vi "lvlib_copy.vi"(7 "configuration":T1={"project_file"="", "lvlibp_directory"="", "zip_directory"="", "lvlib_directory"="", "update_version_vi"="", "installer_post_file"="", "distribution_folder"="", "dependencies_folder"="", "version"="", "bin_folder"="", "lvlib_post_action"=0, "installer_post_action"=0, "application_post_action"=0, "zip_post_action"=1}, 8 "error in (no error)":errorcluster, 11 "library_path":path) -> (0 "error out":errorcluster, 3 "copied_library_path":path)   [LabVIEW 2015, in "lv-builder-default.lvlib"]
uses:
  lv-builder-default.lvlib
  public/_controls/configuration.ctl
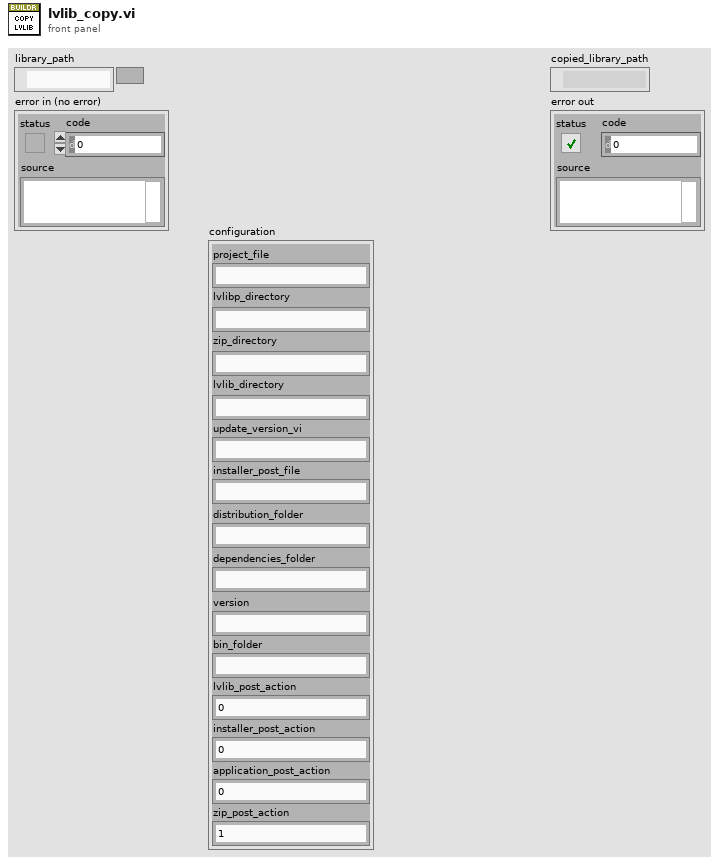
[diagram p1: front panel]
types:
  T1 = typedef "lv-builder-default.lvlib/configuration.ctl" = cluster{"project_file":string, "lvlibp_directory":string, "zip_directory":string, "lvlib_directory":string, "update_version_vi":string, "installer_post_file":string, "distribution_folder":string, "dependencies_folder":string, "version":string, "bin_folder":string, "lvlib_post_action":u16, "installer_post_action":u16, "application_post_action":u16, "zip_post_action":u16}
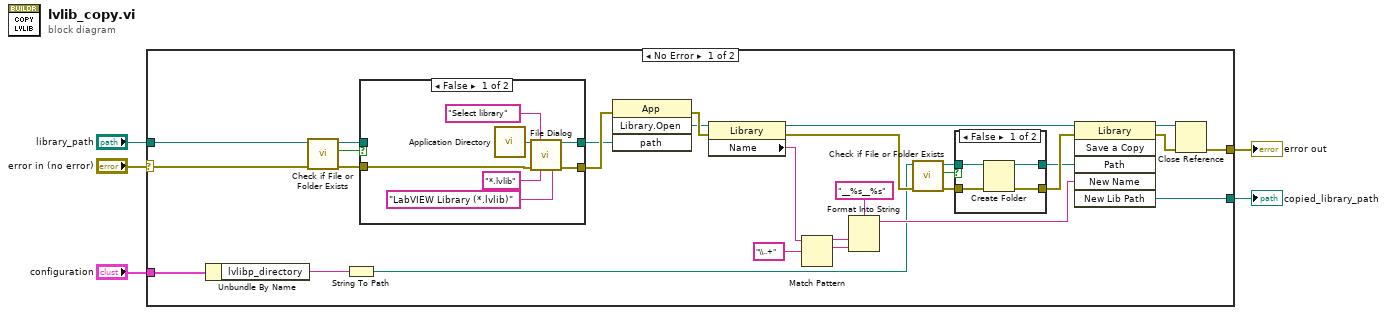
[diagram p0: block diagram]
diagram:
  n1 = case shown="No Error" "error in (no error)" {
    selector: "error in (no error)" -> [w18 w50]
    tunnel: [w21 _] -> w5
    tunnel: [w20 w50] -> w4
    tunnel: "library_path" -> [w19 _]
    tunnel: "configuration" -> [w8 _]
    frame No Error {
      n2 = Unbundle By Name(w8) -> ("lvlibp_directory"=w7:string)
      n3 = call <vilib>:"Check if File or Folder Exists.vi"("error in (no error)"=w18, "path"=w19) -> ("error out"=w17:errorcluster, "file or folder exists?"=w15:bool, "dup path"=w14:path)  [unwired: 7 in]
      n4 = String To Path(string=w7) -> (path=w6:path)
      n5 = case shown="False" w15 {
        tunnel: w17 -> [w43 w48]
        tunnel: [w42 w48] -> w16
        tunnel: w14 -> [_ w49]
        tunnel: [w41 w49] -> w13
        frame False {
          n6 = call <vilib>:"Application Directory.vi"() -> ("Application Directory"=w44:path)
          n7 = call "File Dialog"("start path"=w44, "prompt"="Select library", "error in"=w43, "pattern (all files)"="*.lvlib", "pattern label"="LabVIEW Library (*.lvlib)") -> ("selected path"=w41:path, "error out"=w42:errorcluster)  [unwired: 7 in, 2 out]
        }
        frame True {
        }
      }
      n8 = invoke class="App" method="Library.Open"(error in=w16, "path"=w13) -> (error out=w32:errorcluster, "Open Library"=w31:refnum<vi>)  [unwired: 2 in, 2 out]
      n9 = property class="Library"(reference=w31, error in=w32) -> (reference out=w25:refnum<vi>, error out=w34:errorcluster, "Name"=w30:string)
      n10 = Match Pattern(string=w30, regular expression="\\..+") -> (before substring=w27:string, match substring=w26:string)  [unwired: 1 in, 2 out]
      n11 = Format Into String(format string="__%s__%s", w27, w26) -> (resulting string=w24:string)  [unwired: 2 in, 1 out]
      n12 = call <vilib>:"Check if File or Folder Exists.vi"("error in (no error)"=w34, "path"=w6) -> ("error out"=w11:errorcluster, "file or folder exists?"=w12:bool, "dup path"=w10:path)  [unwired: 7 in]
      n13 = case shown="False" w12 {
        tunnel: w11 -> [w38 w39]
        tunnel: w10 -> [w37 w40]
        tunnel: [w36 w39] -> w33
        tunnel: [w35 w40] -> w9
        frame False {
          n14 = Create Folder(path (use dialog)=w37, error in=w38) -> (created path=w35:path, error out=w36:errorcluster)  [unwired: 1 in, 1 out]
        }
        frame True {
        }
      }
      n15 = invoke class="Library" method="Save a Copy"(reference=w25, error in=w33, "Path"=w9, "New Name"=w24) -> (reference out=w22:refnum<vi>, error out=w23:errorcluster, "New Lib Path"=w21:path)  [unwired: 2 in, 3 out]
      n16 = Close Reference(reference=w22, error in (no error)=w23) -> (error out=w20:errorcluster)
    }
    frame Error {
    }
  }
  "copied_library_path" <- w5
  "error out" <- w4
